vi "get Live.vi"(10 "live":u64, 11 "devID":u32) -> (2 "live out":u64, 3 "function return":i32)   [LabVIEW 2014, in "libchaos-driver-powersupply-labview.lvlib"]
doc: "int getLive(unsigned int devID,long long *live);"
uses:
  libchaos-driver-powersupply-labview.lvlib
  chaos-i686-dynamic-release/lib/libchaos-driver-powersupply-labview.so
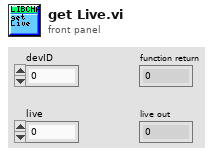
[diagram p1: front panel]
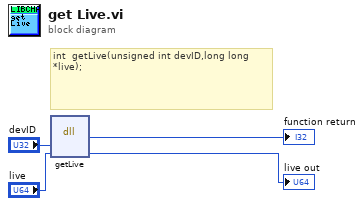
[diagram p0: block diagram]
diagram:
  # "int  getLive(unsigned int devID,long long *live);"
  n1 = dll-call lib="home/chaos/chaos_bundle/chaos-i686-dynamic-release/lib/libchaos-driver-powersupply-labview.*" fn="getLive"("devID"="devID", "live"="live") -> (→"function return":i32, "live"=→"live out":u64)  [unwired: 4 in, 2 out]
